vi "Routine.Create.vi"(8 "error in (no error)":errorcluster, 10 "Routine":T1 {"Stop Parameters"."Response"."Byte Order" items=["Little Endian", "Big Endian"]; "Stop Parameters"."Response"."Data Type" items=["Signed", "Unsigned", "IEEE Float"]; "Stop Parameters"."Cmd"."Byte Order" items=["Little Endian", "Big Endian"]; "Stop Parameters"."Cmd"."Data Type" items=["Signed", "Unsigned", "IEEE Float"]; "Request Parameters"."Response"."Byte Order" items=["Little Endian", "Big Endian"]; "Request Parameters"."Response"."Data Type" items=["Signed", "Unsigned", "IEEE Float"]; "Request Parameters"."Cmd"."Byte Order" items=["Little Endian", "Big Endian"]; "Request Parameters"."Cmd"."Data Type" items=["Signed", "Unsigned", "IEEE Float"]; "Start Parameters"."Response"."Byte Order" items=["Little Endian", "Big Endian"]; "Start Parameters"."Response"."Data Type" items=["Signed", "Unsigned", "IEEE Float"]; "Start Parameters"."Cmd"."Byte Order" items=["Little Endian", "Big Endian"]; "Start Parameters"."Cmd"."Data Type" items=["Signed", "Unsigned", "IEEE Float"]}, 11 "Section Ptr":T4 format="%.0x") -> (0 "error out":errorcluster, 3 "Parent Ref out":T4 format="%.0x")   [LabVIEW 2015, in "Diagnostics Addon System Explorer.lvlib"]
uses:
  Diagnostics Addon System Explorer.lvlib
  <vilib>/NI Veristand/Custom Device API/Custom Device Item Ref.ctl
  Types/Routine.Export.ctl
  Types/CmdResp.Export.ctl
  Shared/Types/Signal.ctl
  Types/FG.Action.ctl
  Shared/Types/Type.ctl
  <vilib>/NI Veristand/Custom Device API/NI VeriStand - Get Item Property.vi
  <vilib>/NI Veristand/Custom Device API/Get Item Property (U32).vi
  <vilib>/NI/NIVS System Definition Utilities/SysDef API/SysDef.Property.Set.vi
  <vilib>/NI/NIVS System Definition Utilities/_SubVIs/SysDef.Property.Set.U32.vi
  Shared/SubVIs/Constants.vi
  Shared/Diagnostics Addon Shared.lvlib
  <vilib>/NI/NIVS System Definition Utilities/System Definition Utilities.lvlib
  <vilib>/NI Veristand/Custom Device API/Custom Device API.lvlib
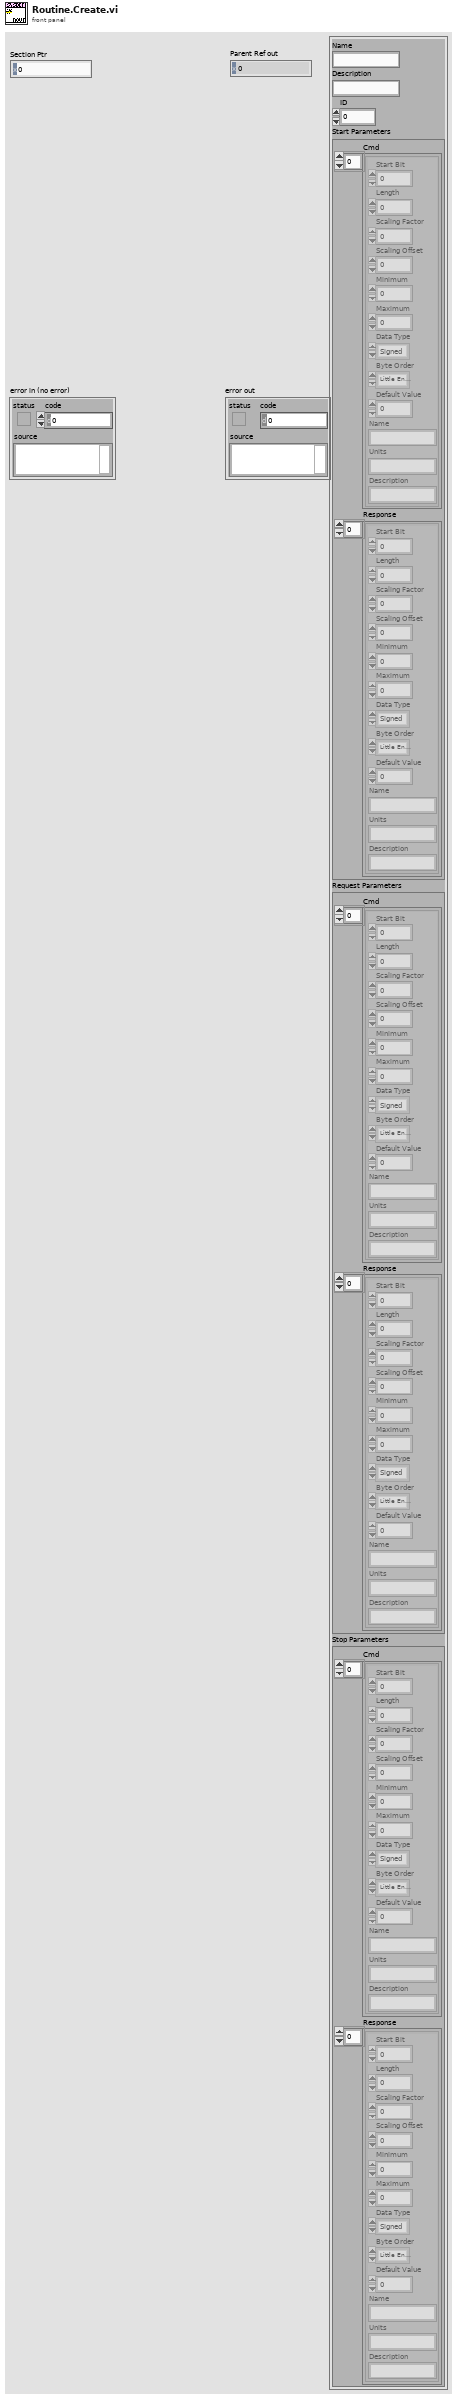
[diagram p1: front panel]
types:
  T1 = typedef "Diagnostics Addon System Explorer.lvlib/Routine.Export.ctl" = cluster{"Name":string, "Description":string, "ID":u16, "Start Parameters":T2, "Request Parameters":T2, "Stop Parameters":T2}
  T2 = typedef "Diagnostics Addon System Explorer.lvlib/CmdResp.Export.ctl" = cluster{"Cmd":T3[], "Response":T3[]}
  T3 = typedef "Diagnostics Addon Shared.lvlib/Signal.ctl" = cluster{"Start Bit":u32, "Length":u32, "Scaling Factor":dbl, "Scaling Offset":dbl, "Minimum":dbl, "Maximum":dbl, "Data Type":u32, "Byte Order":u32, "Default Value":dbl, "Name":string, "Units":string, "Description":string}
  T4 = typedef "Custom Device API.lvlib/Custom Device Item Ref.ctl" = u64
  T5 = typedef "Diagnostics Addon System Explorer.lvlib/FG.Action.ctl" = enum16{"Get", "Set"}
  T6 = typedef "Diagnostics Addon Shared.lvlib/Type.ctl" = enum16{"DID", "CDID", "PID", "CPID", "Read Memory", "Write Memory", "DTC Control", "IO Cmd", "IO Resp", "Routine Start Cmd", "Routine Start Resp", "Routine Request Cmd", "Routine Request Resp", "Routine Stop Cmd", "Routine Stop Resp", "UserDefined Cmd", "UserDefined Rsp"}
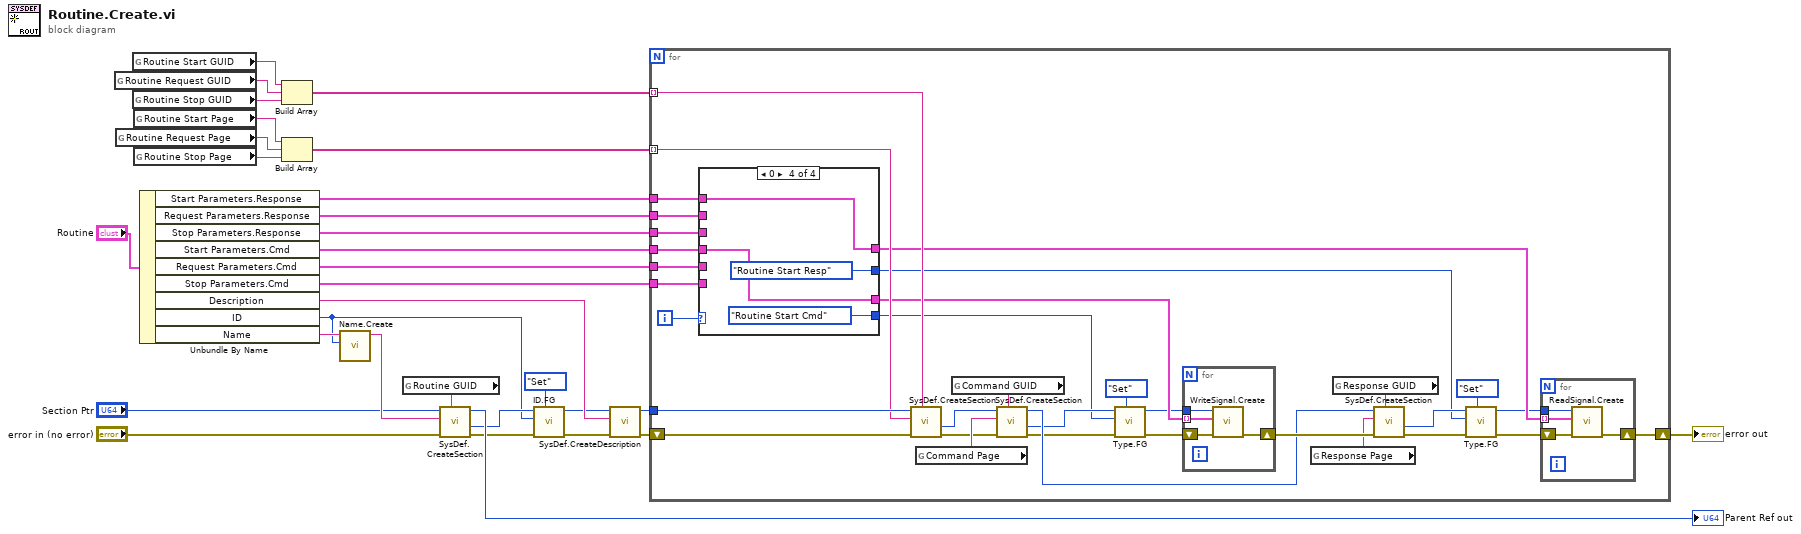
[diagram p0: block diagram]
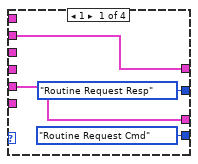
[diagram p2: hidden frame]
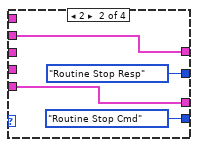
[diagram p3: hidden frame]
diagram:
  n1 = global read "Constants.vi" "Routine Request GUID"() -> (w30:string)
  n2 = global read "Constants.vi" "Routine Request Page"() -> (w26:string)
  n3 = global read "Constants.vi" "Routine Start GUID"() -> (w29:string)
  n4 = global read "Constants.vi" "Routine Stop GUID"() -> (w31:string)
  n5 = global read "Constants.vi" "Routine Start Page"() -> (w27:string)
  n6 = global read "Constants.vi" "Routine Stop Page"() -> (w25:string)
  n7 = Unbundle By Name("Routine") -> ("Start Parameters.Response"=w12:T3[], "Request Parameters.Response"=w10:T3[], "Stop Parameters.Response"=w8:T3[], "Start Parameters.Cmd"=w11:T3[], "Request Parameters.Cmd"=w9:T3[], "Stop Parameters.Cmd"=w7:T3[], "Description"=w20:string, "ID"=w1:u16, "Name"=w21:string)
  n8 = Build Array(w29, w30, w31) -> (w28:string[])
  n9 = Build Array(w27, w26, w25) -> (w24:string[])
  n10 = call "Name.Create.vi"("PID Number"=w1, "PID Name"=w21) -> ("VS Name"=w23:string)  [unwired: 9 in]
  n11 = global read "Constants.vi" "Routine GUID"() -> (w17:string)
  n12 = call <vilib>:"SysDef.CreateSection.vi"("GUID"=w17, "error in (no error)"="error in (no error)", "Name"=w23, "nodeID"="Section Ptr") -> ("error out"=w5:errorcluster, "New NodeID"=w4:u64, "nodeID out"=→"Parent Ref out":u64)  [unwired: 4 in, 1 out]
  n13 = call "ID.FG.vi"("Action"=FG.Action."Set", "error in (no error)"=w5, "ID"=w1, "Device Item Ref in"=w4) -> ("error out"=w3:errorcluster, "Device Item Ref out"=w2:T4)  [unwired: 5 in, 1 out]
  n14 = call <vilib>:"SysDef.CreateDescription.vi"("error in (no error)"=w3, "Description"=w20, "ID in"=w2) -> ("error out"=w19:errorcluster, "ID out"=w18:T4)  [unwired: 7 in]
  n15 = for {
    tunnel: w18 -> [w64]
    shift-right: [w55] -> w14
    shift-left: w19 -> [w65]
    tunnel: w28 -> [w63] mode=indexing
    tunnel: w24 -> [w62] mode=indexing
    tunnel: w12 -> [w50]
    tunnel: w11 -> [w48]
    tunnel: w10 -> [w47]
    tunnel: w9 -> [w46]
    tunnel: w8 -> [w45]
    tunnel: w7 -> [w44]
    i -> [w52]
    n16 = case shown="0" w52 {
      tunnel: [w69 w73 _ w77] -> w51
      tunnel: w50 -> [_ _ _ w77]
      tunnel: [w68 w72 _ w76] -> w49
      tunnel: w48 -> [_ _ _ w76]
      tunnel: w47 -> [w69 _ _ _]
      tunnel: w46 -> [w68 _ _ _]
      tunnel: w45 -> [_ w73 _ _]
      tunnel: w44 -> [_ w72 _ _]
      tunnel: [Type."Routine Request Cmd" ("CmdType") Type."Routine Stop Cmd" ("CmdType") _ Type."Routine Start Cmd" ("CmdType")] -> w33
      tunnel: [Type."Routine Request Resp" ("RespType") Type."Routine Stop Resp" ("RespType") _ Type."Routine Start Resp" ("RespType")] -> w32
      frame 1 {
      }
      frame 2 {
      }
      frame Default {
      }
      frame 0 {
      }
    }
    n17 = call <vilib>:"SysDef.CreateSection.vi"("GUID"=w63, "error in (no error)"=w65, "Name"=w62, "nodeID"=w64) -> ("error out"=w54:errorcluster, "New NodeID"=w53:u64)  [unwired: 4 in, 2 out]
    n18 = global read "Constants.vi" "Command Page"() -> (w56:string)
    n19 = global read "Constants.vi" "Command GUID"() -> (w57:string)
    n20 = call <vilib>:"SysDef.CreateSection.vi"("GUID"=w57, "error in (no error)"=w54, "Name"=w56, "nodeID"=w53) -> ("error out"=w41:errorcluster, "New NodeID"=w39:u64, "nodeID out"=w60:u64)  [unwired: 4 in, 1 out]
    n21 = call "Type.FG.vi"("Action"=FG.Action."Set", "error in (no error)"=w41, "Type"=w33, "Device Item Ref in"=w39) -> ("error out"=w40:errorcluster, "Device Item Ref out"=w38:T4)  [unwired: 5 in, 1 out]
    n22 = for {
      shift-right: [w80] -> w61
      shift-left: w40 -> [w81]
      tunnel: w49 -> [w79] mode=indexing
      tunnel: w38 -> [w78]
      n23 = call "WriteSignal.Create.vi"("error in (no error)"=w81, "Signal Parameters"=w79, "Section Ptr"=w78) -> ("error out"=w80:errorcluster)  [unwired: 7 in, 1 out]
    }
    n24 = global read "Constants.vi" "Response Page"() -> (w59:string)
    n25 = global read "Constants.vi" "Response GUID"() -> (w58:string)
    n26 = call <vilib>:"SysDef.CreateSection.vi"("GUID"=w58, "error in (no error)"=w61, "Name"=w59, "nodeID"=w60) -> ("error out"=w37:errorcluster, "New NodeID"=w35:u64)  [unwired: 4 in, 2 out]
    n27 = call "Type.FG.vi"("Action"=FG.Action."Set", "error in (no error)"=w37, "Type"=w32, "Device Item Ref in"=w35) -> ("error out"=w36:errorcluster, "Device Item Ref out"=w34:T4)  [unwired: 5 in, 1 out]
    n28 = for {
      shift-right: [w84] -> w55
      shift-left: w36 -> [w85]
      tunnel: w51 -> [w83] mode=indexing
      tunnel: w34 -> [w82]
      n29 = call "ReadSignal.Create.vi"("error in (no error)"=w85, "Signal Parameters"=w83, "Section Ptr"=w82) -> ("error out"=w84:errorcluster)  [unwired: 7 in, 1 out]
    }
  }
  "error out" <- w14
